vi "example_batchAlignment.vi"() -> ()   [LabVIEW 2023]
uses:
  <vilib>/numeric/Random Number (Range) U64.vi
  <vilib>/numeric/sub_Random U32.vi
panel:
  in  "alignHorizontalCenters":bool
  in  "alignVerticalCenters":bool
  in  "alignBottom":bool
  in  "alignTop":bool
  in  "useControlBodyOnly":bool=TRUE caption="Use Control Body Only\n(=ignore labels & captions)"
  in  "stop":bool
  in  "alignRight":bool
  in  "alignLeft":bool
  in  "shuffle":bool
  in  "control 3":string
  in  "control 2":bool
  in  "control 1":string
  in  "control 0":dbl
  # "Instruction:\n1. Press Shuffle button to place the target objects randomly.\n2. Press the Alignment button you prefer."
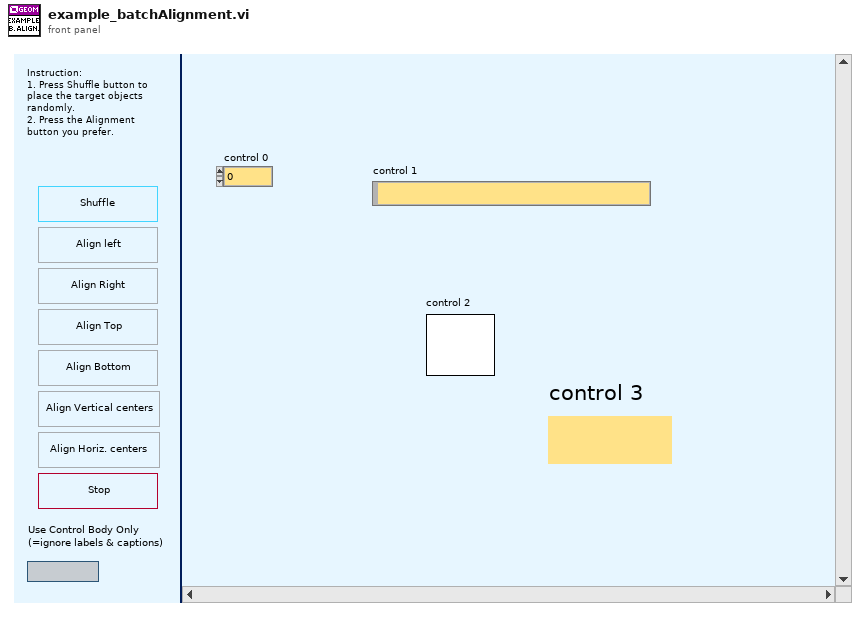
[diagram p1: front panel]
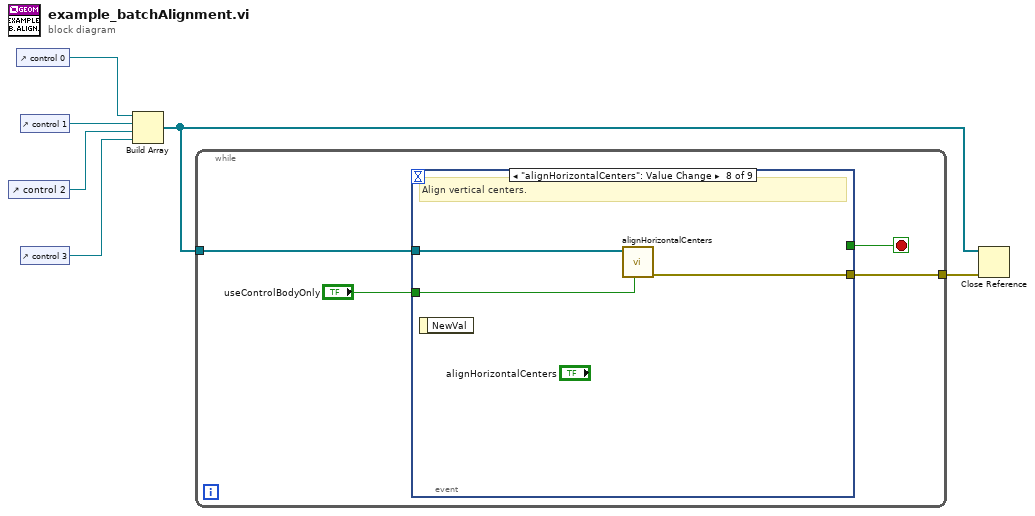
[diagram p0: block diagram]
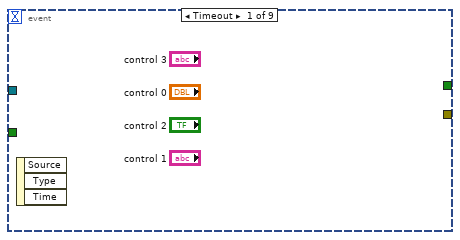
[diagram p2: hidden frame]
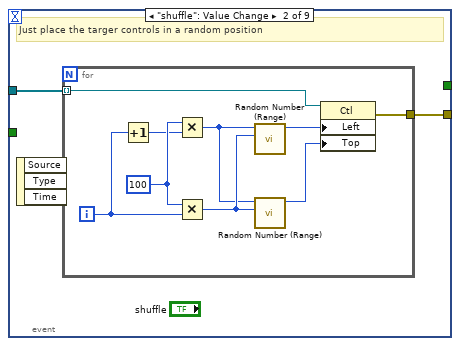
[diagram p3: hidden frame]
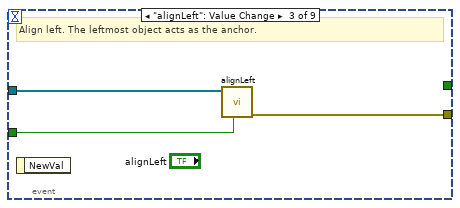
[diagram p4: hidden frame]
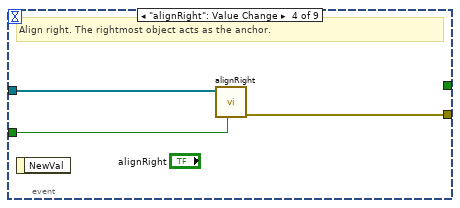
[diagram p5: hidden frame]
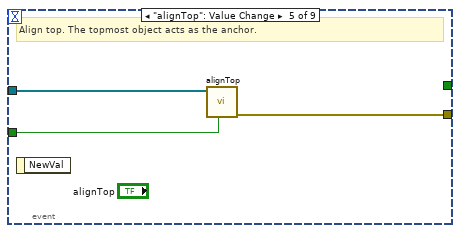
[diagram p6: hidden frame]
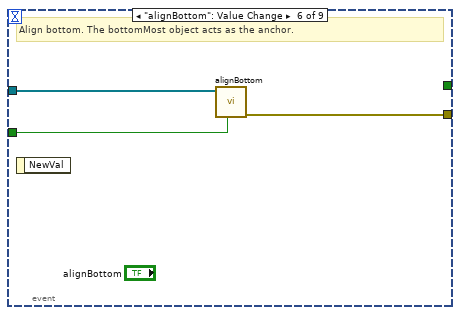
[diagram p7: hidden frame]
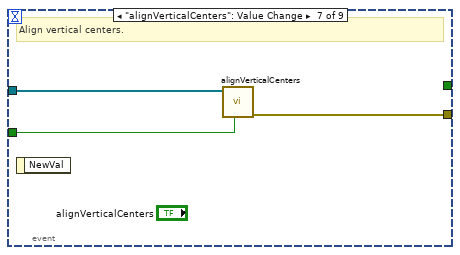
[diagram p8: hidden frame]
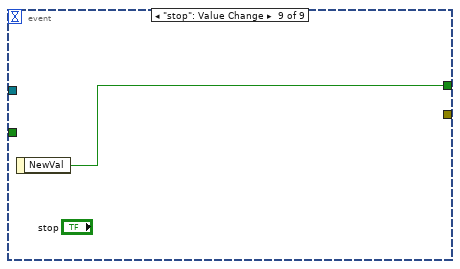
[diagram p9: hidden frame]
diagram:
  n1 = control-ref of="control 2"() -> (w5:refnum<vi>)
  n2 = control-ref of="control 0"() -> (w1:refnum<vi>)
  n3 = control-ref of="control 1"() -> (w6:refnum<vi>)
  n4 = control-ref of="control 3"() -> (w4:refnum<vi>)
  n5 = Build Array(w1, w6, w5, w4) -> (w3:refnum<vi>[])
  n6 = while {
    tunnel: w3 -> [w9]
    tunnel: [w8] -> w2
    stop <- w10 stop-if-true
    n7 = event shown="[7] \"alignHorizontalCenters\": Value Change" {
      selector: _ -> [_ _ _ _ _ _ _ _ _]
      dyn-events: _ -> [_ _ _ _ _ _ _ _ _]
      timeout: _ -> [_ _ _ _ _ _ _ _ _]
      tunnel: [_ _ _ _ _ _ _ _ w40] -> w10
      tunnel: w9 -> [_ w12 w24 w27 w30 w33 w36 w39 _]
      tunnel: [_ w11 w22 w25 w28 w31 w34 w37 _] -> w8
      tunnel: "useControlBodyOnly" -> [_ _ w23 w26 w29 w32 w35 w38 _]
      event Timeout {
        n8 = event-data() -> ()  [unwired: 1 in, 3 out]
      }
      event "shuffle": Value Change {
        # "Just place the targer controls in a random position"
        n9 = event-data() -> ()  [unwired: 1 in, 3 out]
        n10 = for {
          tunnel: w12 -> [w21] mode=indexing
          tunnel: [w18] -> w11
          i -> [w17]
          w16 = u64 100 ("upper bound (100)")
          n11 = Increment(x=w17) -> (x+1=w14:i32)
          n12 = Multiply(x=w16, y=w14) -> (x*y=w13:u64)
          n13 = Multiply(x=w16, y=w17) -> (x*y=w15:u64)
          n14 = call-poly <vilib>:"Random Number (Range).vi"("lower bound (0)"=w15, "upper bound (100)"=w13) -> ("number"=w20:u64)  [unwired: 9 in]
          n15 = call-poly <vilib>:"Random Number (Range).vi"("lower bound (0)"=w15, "upper bound (100)"=w13) -> ("number"=w19:u64)  [unwired: 9 in]
          n16 = property class="Ctl"(reference=w21, "Left"=w20, "Top"=w19) -> (error out=w18:errorcluster)  [unwired: 1 in, 1 out]
        }
      }
      event "alignLeft": Value Change {
        # "Align left. The leftmost object acts as the anchor."
        n17 = event-data() -> ()  [unwired: 1 in, 1 out]
        n18 = call "alignLeft.vi"("useControlBodyOnly"=w23, "refs"=w24) -> ("error out"=w22:errorcluster)  [unwired: 8 in, 1 out]
      }
      event "alignRight": Value Change {
        # "Align right. The rightmost object acts as the anchor."
        n19 = event-data() -> ()  [unwired: 1 in, 1 out]
        n20 = call "alignRight.vi"("useControlBodyOnly"=w26, "refs"=w27) -> ("error out"=w25:errorcluster)  [unwired: 8 in, 1 out]
      }
      event "alignTop": Value Change {
        # "Align top. The topmost object acts as the anchor."
        n21 = event-data() -> ()  [unwired: 1 in, 1 out]
        n22 = call "alignTop.vi"("useControlBodyOnly"=w29, "refs"=w30) -> ("error out"=w28:errorcluster)  [unwired: 8 in, 1 out]
      }
      event "alignBottom": Value Change {
        # "Align bottom. The bottomMost object acts as the anchor."
        n23 = event-data() -> ()  [unwired: 1 in, 1 out]
        n24 = call "alignBottom.vi"("useControlBodyOnly"=w32, "refs"=w33) -> ("error out"=w31:errorcluster)  [unwired: 8 in, 1 out]
      }
      event "alignVerticalCenters": Value Change {
        # "Align vertical centers."
        n25 = event-data() -> ()  [unwired: 1 in, 1 out]
        n26 = call "alignVerticalCenters.vi"("useControlBodyOnly"=w35, "refs"=w36) -> ("error out"=w34:errorcluster)  [unwired: 8 in, 1 out]
      }
      event "alignHorizontalCenters": Value Change {
        # "Align vertical centers."
        n27 = event-data() -> ()  [unwired: 1 in, 1 out]
        n28 = call "alignHorizontalCenters.vi"("useControlBodyOnly"=w38, "refs"=w39) -> ("error out"=w37:errorcluster)  [unwired: 8 in, 1 out]
      }
      event "stop": Value Change {
        n29 = event-data() -> ("NewVal"=w40:bool)  [unwired: 1 in]
      }
    }
  }
  n30 = Close Reference(reference=w3, error in (no error)=w2) -> ()  [unwired: 1 out]
